vi "Pump.vi"(6 "deadline":T1={"mode"=enum."Relative", "deadline (ms)"=30000}, 8 "error in (no error)":errorcluster, 11 "subprocess in":refnum<class "Buffered Subprocess.lvclass">) -> (0 "error out":errorcluster, 3 "subprocess out":refnum<class "Buffered Subprocess.lvclass">)   [LabVIEW 2020, in "NI_Subprocess.lvlib" / "Buffered Subprocess.lvclass"]
uses:
  <vilib>/Subprocess/Buffered Subprocess/Buffered Subprocess.lvclass
  <vilib>/Utility/Deadline/Deadline.ctl
  <vilib>/Utility/Deadline/Mode.ctl
  <vilib>/Subprocess/Buffered Subprocess/Buffered Subprocess.lvclass/Buffered Subprocess.ctl
  <vilib>/Array/Bytestream/Bytestream.lvclass/Bytestream.ctl
  7f63ec14-092a-3fee-b81b-f224ecbece3f.vi
  f38d2210-e546-3fd6-f096-0bc968b0c23f.vi
  <vilib>/Array/Bytestream/Get Logical Datum.vi
  <vilib>/Array/Bytestream/Datum Size.vi
  <vilib>/Array/Bytestream/Count Datums.vi
  <vilib>/Array/Bytestream/Append.vi
  <vilib>/Array/Bytestream/Grow If Necessary.vi
  <vilib>/Array/Bytestream/Next Available Datum Index.vi
  <vilib>/Array/Bytestream/Count Allocated Datums.vi
  <vilib>/Array/Bytestream/Grow Datum Array.vi
  <vilib>/Utility/error.llb/Error Cluster From Error Code.vi
  <vilib>/Array/Bytestream/Bytestream.lvclass
  <vilib>/ErrorRing/Error Ring.xnode
  <vilib>/Subprocess/Subprocess/Subprocess.lvclass
  <vilib>/Utility/Deadline/NI_Deadline.lvlib
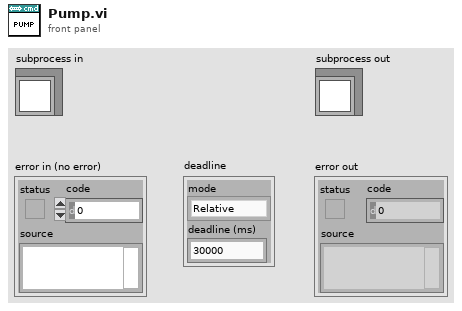
[diagram p1: front panel]
types:
  T1 = typedef "NI_Deadline.lvlib/Deadline.ctl" = cluster{"mode":T2, "deadline (ms)":u32}
  T2 = typedef "NI_Deadline.lvlib/Mode.ctl" = enum16{"Relative", "Use deadline", "Wait forever", "Nonblocking", "N/A"}
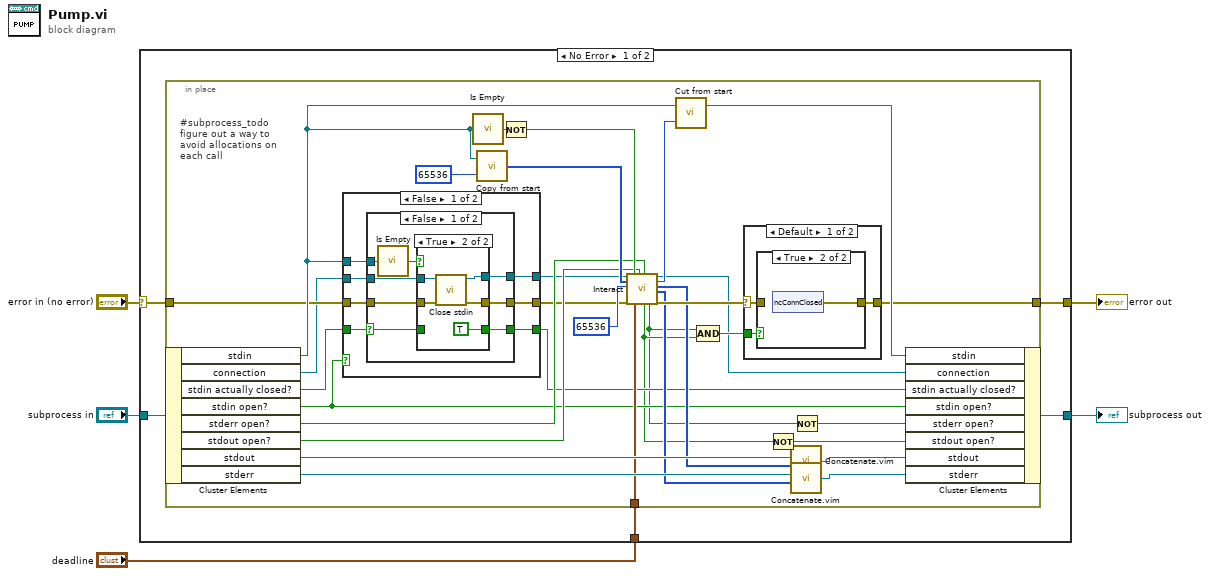
[diagram p0: block diagram]
diagram:
  n1 = case shown="No Error" "error in (no error)" {
    selector: "error in (no error)" -> [w10 w83]
    tunnel: [w6 w83] -> w4
    tunnel: "subprocess in" -> [w9 w82]
    tunnel: [w7 w82] -> w2
    tunnel: "deadline" -> [w8 _]
    frame No Error {
      n2 = in-place "In Place Element Structure" {
        in-place-border: w10 -> [w22]
        in-place-border: [w21] -> w6
        in-place-border: w8 -> [w25]
        # "#subprocess_todo figure out a way to avoid allocations on each call"
        n3 = in-place-cluster #1 ("Unbundle / Bundle Elements")(w9) -> ("stdin"=w24:refnum<class "Bytestream.lvclass">, "connection"=w19:refnum<class "Subprocess.lvclass">, "stdin actually closed?"=w17:bool, "stdin open?"=w16:bool, "stderr open?"=w32:bool, "stdout open?"=w31:bool, "stdout"=w37:refnum<class "Bytestream.lvclass">, "stderr"=w36:refnum<class "Bytestream.lvclass">)
        n4 = case shown="False" w16 {
          tunnel: w19 -> [w56 w81]
          tunnel: w22 -> [w57 w80]
          tunnel: w24 -> [w58 _]
          tunnel: w17 -> [w59 w79]
          tunnel: [w55 w81] -> w20
          tunnel: [w54 w80] -> w23
          tunnel: [w53 w79] -> w15
          frame False {
            n5 = case shown="False" w59 {
              selector: w59 -> [w61 w78]
              tunnel: w58 -> [w67 _]
              tunnel: w57 -> [w66 w76]
              tunnel: w56 -> [w65 w77]
              tunnel: [w64 w77] -> w55
              tunnel: [w63 w76] -> w54
              tunnel: [w62 w78] -> w53
              frame False {
                n6 = call <vilib>:"Is Empty.vi"("a"=w67) -> ("empty?"=w60:bool)
                n7 = case shown="True" w60 {
                  tunnel: w66 -> [w69 w74]
                  tunnel: w65 -> [w68 w75]
                  tunnel: [w68 w73] -> w64
                  tunnel: [w69 w72] -> w63
                  tunnel: [w70 TRUE] -> w62
                  tunnel: w61 -> [w70 _]
                  frame False {
                  }
                  frame True {
                    n8 = call <vilib>:"Close stdin.vi"("error in (no error)"=w74, "subprocess in"=w75) -> ("error out"=w72:errorcluster, "subprocess out"=w73:refnum<class "Subprocess.lvclass">)  [unwired: 8 in]
                  }
                }
              }
              frame True {
              }
            }
          }
          frame True {
          }
        }
        n9 = call <vilib>:"Is Empty.vi"("a"=w24) -> ("empty?"=w38:bool)
        n10 = call <vilib>:"Copy from start.vi"("length"=65536, "bytestream"=w24) -> ("data"=w39:u8[])
        n11 = Not(x=w38) -> (.not. x?=w40:bool)
        n12 = call <vilib>:"Interact.vi"("subprocess in"=w20, "stdin buffer"=w39, "read size"=65536 ("dimension size"), "error in"=w23, "select stdin"=w40, "deadline"=w25, "select stdout"=w31, "select stderr"=w32) -> ("stdout eof?"=w14:bool, "stderr eof?"=w12:bool, "subprocess out"=w18:refnum<class "Subprocess.lvclass">, "stdin written"=w42:i32, "stdout buffer out"=w27:u8[], "stderr buffer out"=w26:u8[], "error out"=w29:errorcluster)  [unwired: 5 in]
        n13 = call <vilib>:"Cut from start.vi"("bytes to cut"=w42, "bytestream in"=w24) -> ("bytestream out"=w30:refnum<class "Bytestream.lvclass">)  [unwired: 1 out]
        n14 = Compound Arithmetic op=AND(w12, w14) -> (w28:bool)
        n15 = case shown="Default" w29 {
          selector: w29 -> [w45 w52]
          tunnel: w28 -> [w43 _]
          tunnel: [w44 w52] -> w21
          frame #0 {
            n16 = case shown="True" w43 {
              tunnel: w45 -> [w46 _]
              tunnel: [w46 w47] -> w44
              frame False {
              }
              frame True {
                n17 = xnode "ncConnClosed"() -> ("error out"=w47:errorcluster)
              }
            }
          }
          frame #1 {
          }
        }
        n18 = Not(x=w14) -> (.not. x?=w13:bool)
        n19 = call "Concatenate.vim"("b"=w27, "a"=w37) -> ("a+b"=w35:refnum<class "Bytestream.lvclass">)  [unwired: 2 in]
        n20 = call "Concatenate.vim"("b"=w26, "a"=w36) -> ("a+b"=w34:refnum<class "Bytestream.lvclass">)  [unwired: 2 in]
        n21 = Not(x=w12) -> (.not. x?=w11:bool)
        n22 = in-place-cluster #1 ("Unbundle / Bundle Elements")("stdin"=w30, "connection"=w18, "stdin actually closed?"=w15, "stdin open?"=w16, "stderr open?"=w11, "stdout open?"=w13, "stdout"=w35, "stderr"=w34) -> (w7:refnum<class "Buffered Subprocess.lvclass">)
      }
    }
    frame Error {
    }
  }
  "error out" <- w4
  "subprocess out" <- w2
